vi "Start Post Processing.vi"(8 "error in (no error)":errorcluster, 10 "Result in":refnum<class "Acquired Result.lvclass">, 11 "Monitor-Pulse in":refnum<class "Monitor-Pulse.lvclass">) -> (0 "error out":errorcluster, 3 "Monitor-Pulse out":refnum<class "Monitor-Pulse.lvclass">)   [LabVIEW 2015, in "Monitor-Pulse.lvclass"]
uses:
  Monitor-Pulse.lvclass
  Measure_core/Results/Acquired Result/Acquired Result.lvclass
  Monitor-Pulse.lvclass/Monitor-Pulse.ctl
  NHMFL_Core/Libraries/Queued Listbox/Queued Listbox.xctl
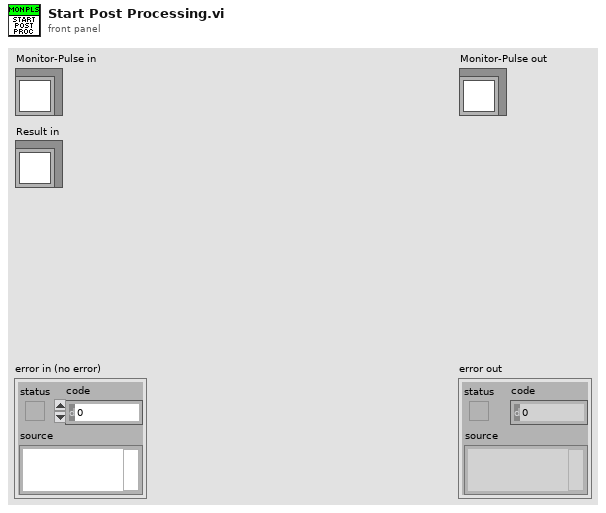
[diagram p1: front panel]
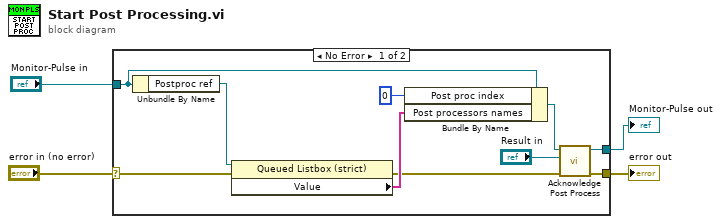
[diagram p0: block diagram]
diagram:
  n1 = case shown="No Error" "error in (no error)" {
    selector: "error in (no error)" -> [w11 w16]
    tunnel: [w6 w16] -> w3
    tunnel: [w5 w15] -> w1
    tunnel: "Monitor-Pulse in" -> [w13 w15]
    frame No Error {
      n2 = Unbundle By Name(w13) -> ("Postproc ref"=w14:refnum<vi>)
      n3 = property class="Queued Listbox (strict)"(reference=w14, error in=w11) -> (error out=w7:errorcluster, "Value"=w12:string[])  [unwired: 1 out]
      n4 = Bundle By Name(cluster=w13, "Post proc index"=0, "Post processors names"=w12) -> (w9:refnum<class "Monitor-Pulse.lvclass">)
      n5 = call-dynamic "Acknowledge Post Process.vi"("error in (no error)"=w7, "Ack Result"="Result in", "Monitor-Pulse in"=w9) -> ("error out"=w6:errorcluster, "Monitor-Pulse out"=w5:refnum<class "Monitor-Pulse.lvclass">)  [unwired: 7 in]
    }
    frame Error {
    }
  }
  "error out" <- w3
  "Monitor-Pulse out" <- w1
